vi "Standard Event Status Query.vi"(0 "VISA resource name":refnum<visa-resource-name>, 11 "error in (no error)":errorcluster) -> (4 "VISA resource name out":refnum<visa-resource-name>, 6 "Standard Event Status Enable":T1, 15 "error out":errorcluster)   [LabVIEW 2014, in "Associated Power Technologies 8500 Series.lvlib"]
doc: "Returns the byte data explaining the events for which the status is being monitored in the instrument.\n\nThe Standard Event Register consists of the following 8 bits.\nBit 0: Operation Complete\nBit 1: not used\nBit 2: Query Error \nBit 3: Device Error\nBit 4: Message Available\nBit 5: Command Error \nBit 6: not used\nBit 7: Power On\n\nExample:\nIf the query gives 0|dec (whose binary equivalent is 00000000|bin) to this VI, no event status will be enabled.\n\nIf 255|dec (11111111|bin) is given, all the events (Operation Complete, User Defined, Query Error, Device Error, Message Available, Command Error,User Defined, Power On) will be enabled."
uses:
  <instrlib>/Associated Power Technologies 8500 Series/Associated Power Technologies 8500 Series.lvlib
panel:
  # "Bit 0: Operation Complete\nBit 1:  not used\nBit 2:  Query Error\t\nBit 3:  Device Error\nBit 4:\t\tMessage Available\nBit 5:  \tCommand Error\t\nBit 6:  not used\nBit 7:  Power On"
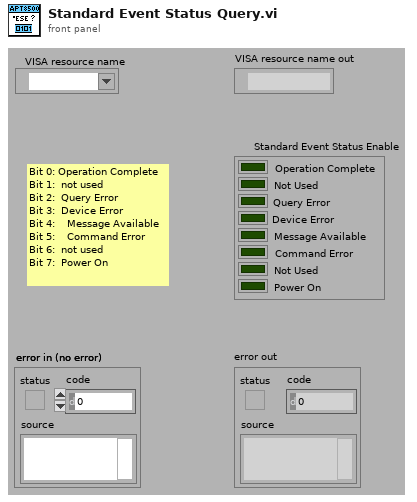
[diagram p1: front panel]
types:
  T1 = cluster{"Operation Complete":bool, "Not Used":bool, "Query Error":bool, "Device Error":bool, "Message Available":bool, "Command Error":bool, "Not Used":bool, "Power On":bool}
  T2 = cluster{"Boolean array[0]":bool, "Boolean array[1]":bool, "Boolean array[2]":bool, "Boolean array[3]":bool, "Boolean array[4]":bool, "Boolean array[5]":bool, "Boolean array[6]":bool, "Boolean array[7]":bool}
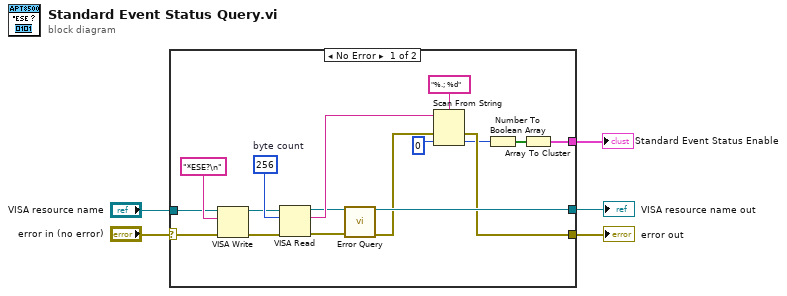
[diagram p0: block diagram]
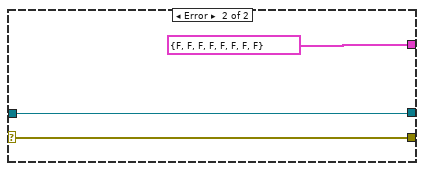
[diagram p2: hidden frame]
diagram:
  n1 = case shown="No Error" "error in (no error)" {
    selector: "error in (no error)" -> [w15 w25]
    tunnel: [w7 w25] -> w5
    tunnel: [w13 w24] -> w4
    tunnel: "VISA resource name" -> [w16 w24]
    tunnel: [w10 T2 {"Boolean array[0]"=FALSE, "Boolean array[1]"=FALSE, "Boolean array[2]"=FALSE, "Boolean array[3]"=FALSE, "Boolean array[4]"=FALSE, "Boolean array[5]"=FALSE, "Boolean array[6]"=FALSE, "Boolean array[7]"=FALSE} ("Boolean array")] -> w1
    frame No Error {
      w21 = u32 256  # byte count
      n2 = VISA Write(VISA resource name=w16, write buffer="*ESE?\n" ("Command to Send (empty)"), error in (no error)=w15) -> (VISA resource name out=w19:refnum<visa-resource-name>, error out=w18:errorcluster)  [unwired: 1 out]
      n3 = VISA Read(VISA resource name=w19, byte count=w21, error in (no error)=w18) -> (VISA resource name out=w12:refnum<visa-resource-name>, read buffer=w20:string, error out=w9:errorcluster)  [unwired: 1 out]
      n4 = call <instrlib>:"Error Query.vi"("VISA resource name"=w12, "error in (no error)"=w9) -> ("VISA resource name out"=w13:refnum<visa-resource-name>, "error out"=w8:errorcluster)  [unwired: 10 in, 2 out]
      n5 = Scan From String(format string="%.; %d" ("Format String"), input string=w20, error in=w8, default 1=u8 0 ("default value 1")) -> (error out=w7:errorcluster, output 1=w6:u8)  [unwired: 1 in, 2 out]
      n6 = Number To Boolean Array(number=w6) -> (Boolean array=w11:bool[])
      n7 = Array To Cluster(array=w11) -> (cluster=w10:T2)
    }
    frame Error {
    }
  }
  "error out" <- w5
  "VISA resource name out" <- w4
  "Standard Event Status Enable" <- w1
